vi "CBR_Player.vi"() -> ()   [LabVIEW 2012]
panel:
  out "text":string
  in  "Vireo":path=path "/Kim/Users/crogers/Documents/LabVIEW Data/LVVIAGenerated/Demo1.vi  2013-12-18 14-09-36.via"
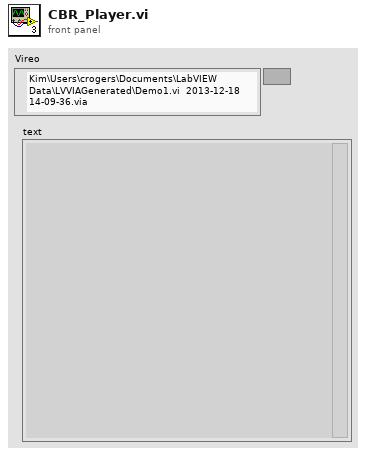
[diagram p1: front panel]
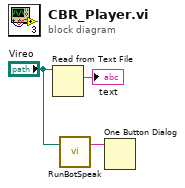
[diagram p0: block diagram]
diagram:
  n1 = Read from Text File(file (use dialog)="Vireo") -> (text=→"text":string)  [unwired: 3 in, 3 out]
  n2 = call <vilib>:"RunBotSpeak.vi"("VIA"="Vireo") -> ("BotSpeak"=w1:string)  [unwired: 2 in]
  n3 = One Button Dialog(message=w1) -> ()  [unwired: 1 in, 1 out]
